vi "Test Case Result Published.vi"(8 "error in (no error)":errorcluster, 11 "Result Observation Test In":refnum<class "Result Observation Test.lvclass">) -> (0 "error out":errorcluster, 3 "Result Observation Test Out":refnum<class "Result Observation Test.lvclass">)   [LabVIEW 2020, in "Result Observation Test.lvclass"]
uses:
  Result Observation Test.lvclass
  C:/Program Files (x86)/National Instruments/LabVIEW 2020/vi.lib/Astemes/LUnit/Test Case.lvclass
  Core/Result/Type.ctl
  Test Case Test Double/Test Case Test Double.lvclass
  C:/Git/astemes-lunit/source/Core/LUnit Test Case/LUnit Test Case V2.lvclass
  <vilib>/Astemes/LUnit/Test Case.lvclass/Test Case.ctl
  <vilib>/Astemes/LUnit/Set Assertion Type.vi
  <vilib>/Astemes/LUnit/Palette/Pass.vi
  <vilib>/Astemes/LUnit/Palette/Fail.vi
  <vilib>/Astemes/LUnit/Add test result.vi
  <vilib>/Astemes/LUnit/LUnit Record Assertion Result.vi
  <vilib>/Astemes/LUnit/LUnit Aggregate Assertion Results.vi
  <vilib>/Astemes/LUnit/Method Result/LUnit Merge Status.vi
  <vilib>/Astemes/LUnit/LUnit Concatenate result strings.vi
  Mock Result Observer/Mock Result Observer.lvclass
  C:/Git/astemes-lunit/source/Core/Result Observer/Result Observer.lvclass
  Core/LUnit Test Suite/LUnit Test Suite.lvclass
  Result Observation Test.lvclass/Result Observation Test.ctl
  Core/Result/Result.lvlib
  <vilib>/Astemes/LUnit/Test Case.lvclass
  C:/Git/astemes-lunit/source/Tests/Result Observation Test/Result Observation Test.lvclass
  C:/Git/astemes-lunit/source/Core/LUnit Test Case/LUnit Test Case.lvclass
  C:/Git/astemes-lunit/source/Core/Runnable/Runnable.lvclass
  C:/Git/astemes-lunit/source/Tests/Test Case Test Double/Test Case Test Double.lvclass
  C:/Git/astemes-lunit/source/Tests/Mock Result Observer/Mock Result Observer.lvclass
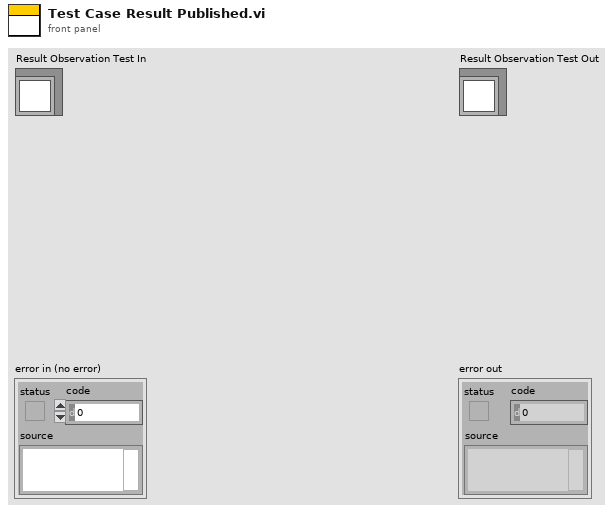
[diagram p1: front panel]
types:
  T1 = typedef "Result.lvlib/Type.ctl" = enum16{"Method", "Case", "Suite", "Pass", "Fail", "Skip", "Pass if", "Fail if", "Pass if Error", "Fail if Error", "Pass if Equal", "Fail if Equal"}
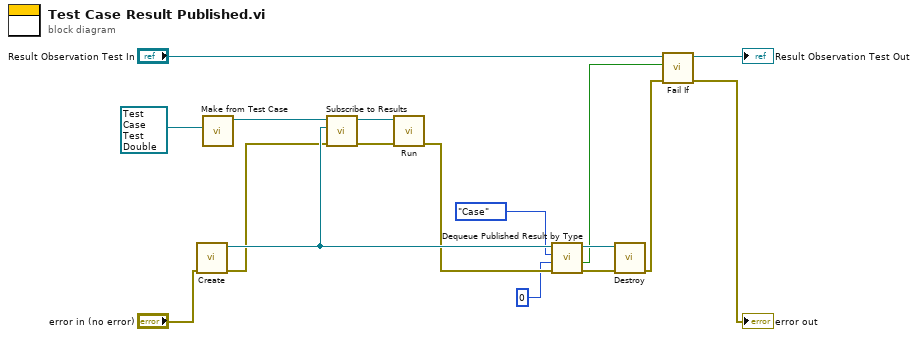
[diagram p0: block diagram]
diagram:
  n1 = call "Create.vi"("error in (no error)"="error in (no error)") -> ("error out"=w1:errorcluster, "Mock Result Observer out"=w13:refnum<class "Mock Result Observer.lvclass">)  [unwired: 9 in]
  n2 = call "Make from Test Case.vi"("LUnit Test Case"=refnum<class "Test Case Test Double.lvclass"> refnum ("LUnit Test Case V2 Test Double.lvclass")) -> ("LUnit Test Suite Out"=w2:refnum<class "LUnit Test Suite.lvclass">)  [unwired: 9 in, 1 out]
  n3 = call-dynamic "Subscribe to Results.vi"("error in (no error)"=w1, "Result Observer"=w13, "LUnit Test Suite In"=w2) -> ("error out"=w10:errorcluster, "LUnit Test Suite Out"=w12:refnum<class "LUnit Test Suite.lvclass">)  [unwired: 7 in]
  n4 = call-dynamic "Run.vi"("error in (no error)"=w10, "LUnit Test Suite In"=w12) -> ("error out"=w9:errorcluster)  [unwired: 8 in, 1 out]
  n5 = call "Dequeue Published Result by Type.vi"("error in (no error)"=w9, "timeout in ms"=0 ("timeout in ms (-1)"), "Result Type"=Type."Case", "Mock Result Observer In"=w13) -> ("error out"=w15:errorcluster, "timed out?"=w6:bool, "Mock Result Observer Out"=w16:refnum<class "Mock Result Observer.lvclass">)  [unwired: 4 in, 1 out]
  n6 = call "Destroy.vi"("error in (no error)"=w15, "Mock Result Observer in"=w16) -> ("error out"=w5:errorcluster)  [unwired: 8 in, 1 out]
  n7 = call <vilib>:"Fail If.vi"("error in (no error)"=w5, "Fail?"=w6, "LUnit Test Case In"="Result Observation Test In") -> ("error out"=→"error out":errorcluster, "LUnit Test Case Out"=→"Result Observation Test Out":refnum<class "Result Observation Test.lvclass">)  [unwired: 7 in]
